vi "Read.vi"(8 "error in (no error)":errorcluster, 11 "Data Class in":refnum<class "Data Class.lvclass">) -> (0 "error out":errorcluster, 1 "Cluster":refnum<class "Cluster.lvclass">, 2 "Class Alias":string, 3 "Data Class out":refnum<class "Data Class.lvclass">)   [LabVIEW 2020, in "Data.lvlib" / "Data Class.lvclass"]
doc: "Read Data Class data."
uses:
  Data Class.lvclass
  Cluster/Cluster.lvclass
  Data Class.lvclass/Data Class.ctl
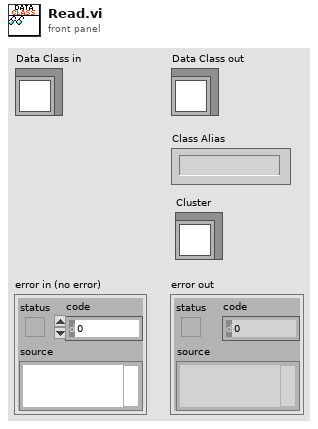
[diagram p1: front panel]
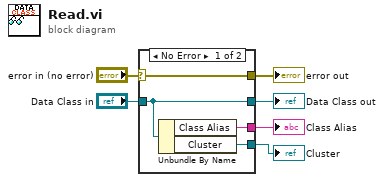
[diagram p0: block diagram]
diagram:
  n1 = case shown="No Error" "error in (no error)" {
    selector: "error in (no error)" -> [w9 w11]
    tunnel: [w9 w11] -> w5
    tunnel: [w10 w12] -> w3
    tunnel: "Data Class in" -> [w10 w12]
    tunnel: [w8 _] -> w2
    tunnel: [w7 _] -> w1
    frame No Error {
      n2 = Unbundle By Name(w10) -> ("Class Alias"=w8:string, "Cluster"=w7:refnum<class "Cluster.lvclass">)
    }
    frame Error {
    }
  }
  "error out" <- w5
  "Data Class out" <- w3
  "Cluster" <- w1
  "Class Alias" <- w2
